vi "swapMotor.vi"(8 "error in (no error)":errorcluster, 10 "Swap motor":bool, 11 "VISA Refnum in":refnum<visa-resource-name>) -> (0 "error out":errorcluster, 3 "VISA Refnum out":refnum<visa-resource-name>)   [LabVIEW 2014]
uses:
  Global Motor Axis.vi
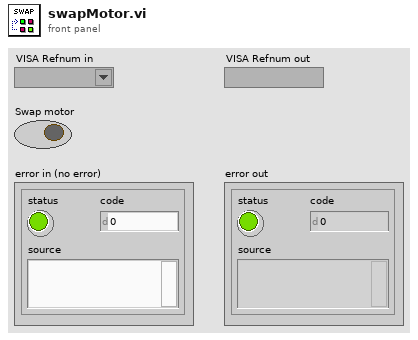
[diagram p1: front panel]
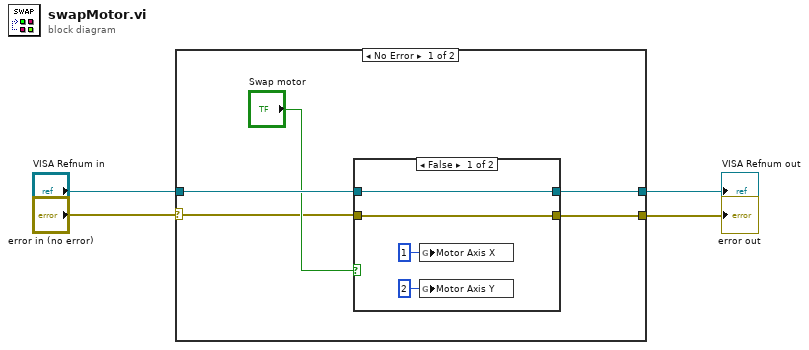
[diagram p0: block diagram]
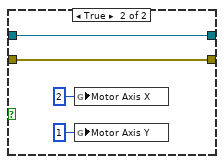
[diagram p2: hidden frame]
diagram:
  n1 = case shown="No Error" "error in (no error)" {
    selector: "error in (no error)" -> [w5 w18]
    tunnel: [w9 w18] -> w4
    tunnel: [w8 w19] -> w3
    tunnel: "VISA Refnum in" -> [w7 w19]
    frame No Error {
      n2 = case shown="False" "Swap motor" {
        tunnel: w7 -> [w11 w15]
        tunnel: w5 -> [w10 w14]
        tunnel: [w11 w15] -> w8
        tunnel: [w10 w14] -> w9
        frame False {
          n3 = global write "Global Motor Axis.vi" "Motor Axis X"(1 ("Motor Axis X")) -> ()
          n4 = global write "Global Motor Axis.vi" "Motor Axis Y"(2 ("Motor Axis Y")) -> ()
        }
        frame True {
          n5 = global write "Global Motor Axis.vi" "Motor Axis X"(2 ("Motor Axis X")) -> ()
          n6 = global write "Global Motor Axis.vi" "Motor Axis Y"(1 ("Motor Axis Y")) -> ()
        }
      }
    }
    frame Error {
    }
  }
  "error out" <- w4
  "VISA Refnum out" <- w3
